vi "Magnet Spec.vi"(3 "Magnet":T2, 7 "Magnet ID":refnum<vi>) -> (0 "min rate (T/min)":dbl, 1 "max rate (T/min)":dbl, 2 "max field (T)":dbl, 4 "max rateS (T/min)":string, 5 "min rateS (T/min)":string, 6 "magnet id":string, 8 "max fieldS (T)":string)   [LabVIEW 2020]
uses:
  Ctl/magnet.ctl
  Ctl/Magnet Spec.ctl
panel:
  in  "Magnet Spec":T1=1
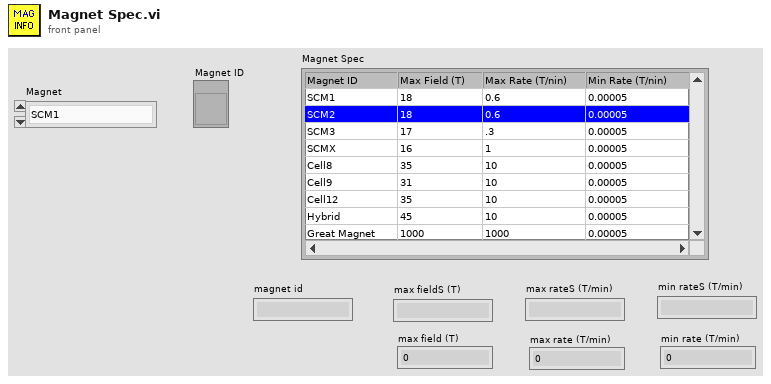
[diagram p1: front panel]
types:
  T1 = typedef "Magnet Spec.ctl" = i32
  T2 = typedef "magnet.ctl" = enum16{"SCM1", "SCM2", "SCM3", "SCMX", "Cell8", "Cell9", "Cell12", "Hybrid", "Great Magnet"}
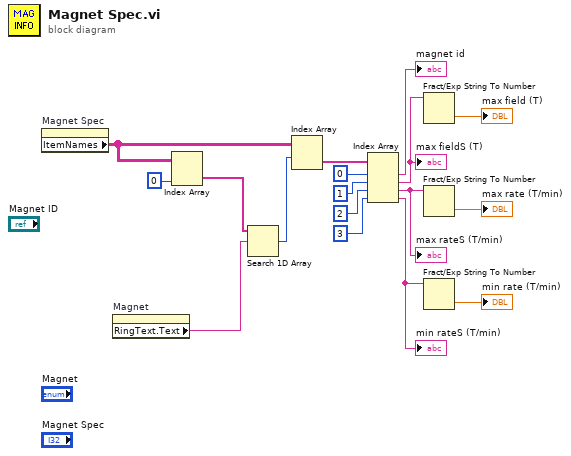
[diagram p0: block diagram]
diagram:
  n1 = property on="Magnet Spec" class="MCListbox (strict)"() -> ("ItemNames"=w9:string[][])  [unwired: 2 in, 2 out]
  n2 = property on="Magnet" class="Enum (strict)"() -> ("RingText.Text"=w1:string)  [unwired: 2 in, 2 out]
  n3 = Index Array(array=w9, index (col)=0 ("disabled index (col)")) -> (element=w16:string[])  [unwired: 1 in]
  n4 = Search 1D Array(1D array=w16, element=w1) -> (index of element=w15:i32)  [unwired: 1 in]
  n5 = Index Array(array=w9, index (row)=w15) -> (element=w14:string[])  [unwired: 1 in]
  n6 = Index Array(array=w14, index #1=0 ("index"), index #2=1 ("index"), index #3=2 ("index"), index #4=3 ("index")) -> (element #1=→"magnet id":string, element #2=w7:string, element #3=w3:string, element #4=w2:string)
  "max fieldS (T)" <- w7
  "max rateS (T/min)" <- w3
  "min rateS (T/min)" <- w2
  n7 = Fract/Exp String To Number(string=w7) -> (number=→"max field (T)":dbl)  [unwired: 3 in, 1 out]
  n8 = Fract/Exp String To Number(string=w3) -> (number=→"max rate (T/min)":dbl)  [unwired: 3 in, 1 out]
  n9 = Fract/Exp String To Number(string=w2) -> (number=→"min rate (T/min)":dbl)  [unwired: 3 in, 1 out]
